vi "Make All Msg.vi"() -> ()   [LabVIEW 2019]
uses:
  00600bcc-c937-488e-a5fa-b30d8be2e7ff.vi
panel:
  out "Horizontal Progress Bar":i32(slide) max=2959 scale=-1.0..1331467.0
  out "size(s)":i32
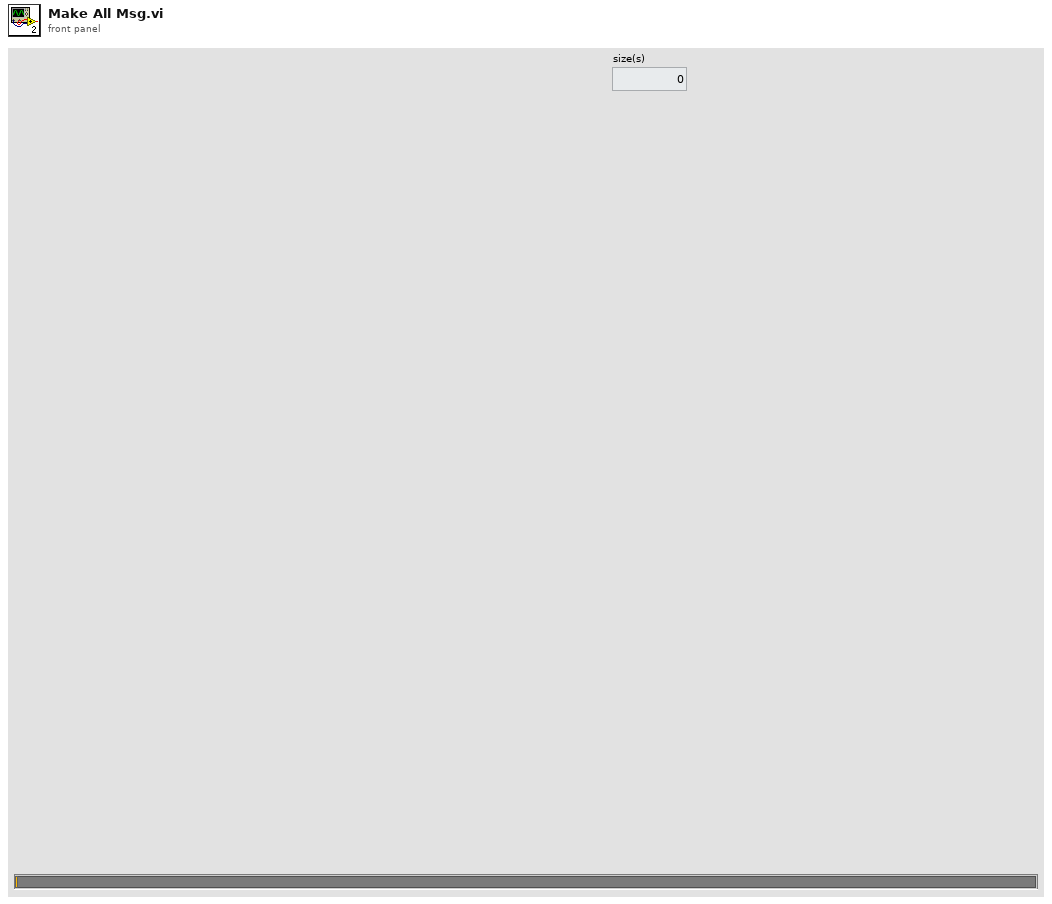
[diagram p1: front panel]
types:
  T1 = enum16{"open", "replace", "create", "open or create", "replace or create", "replace or create with confirmation"}
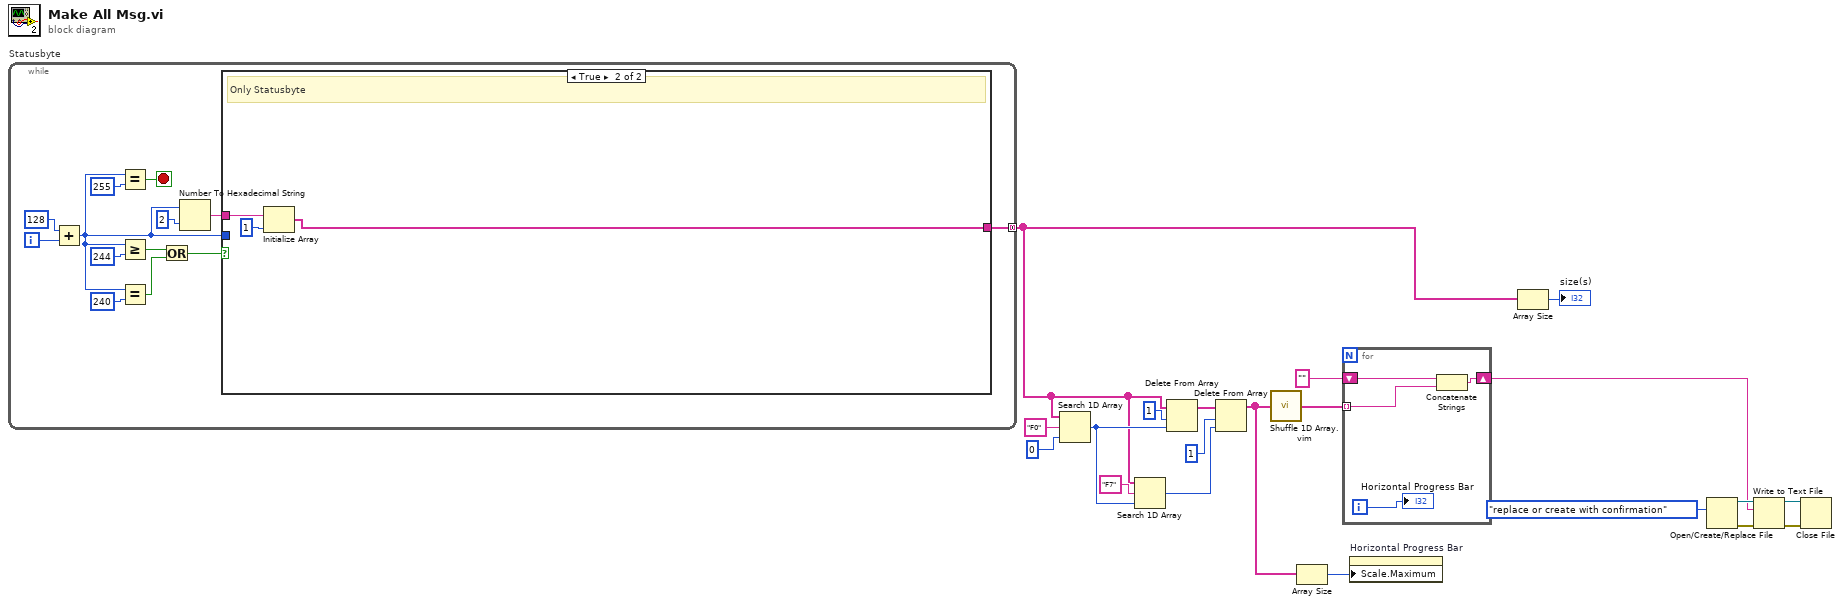
[diagram p0: block diagram]
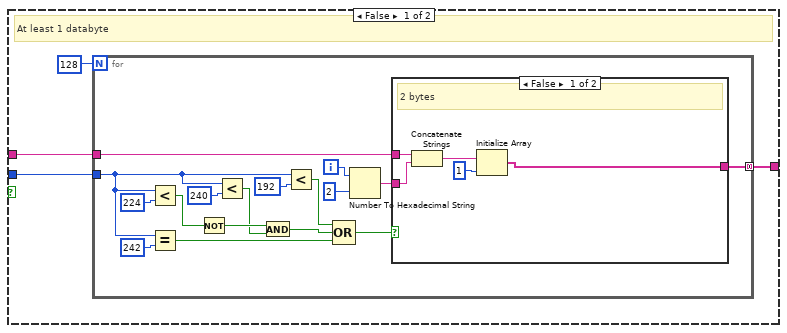
[diagram p2: hidden frame]
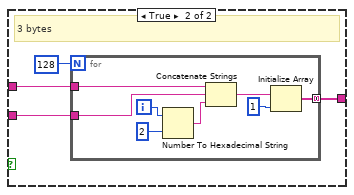
[diagram p3: hidden frame]
diagram:
  n1 = while "Statusbyte" {
    tunnel: [w29] -> w12 mode=concatenating
    i -> [w32]
    stop <- w28 stop-if-true
    n2 = Add(x=128, y=w32) -> (x+y=w23:i32)
    n3 = Equal?(x=w23, y=255) -> (x = y?=w28:bool)
    n4 = Greater Or Equal?(x=w23, y=244) -> (x >= y?=w26:bool)
    n5 = Equal?(x=w23, y=240) -> (x = y?=w21:bool)
    n6 = Or(x=w26, y=w21) -> (x .or. y?=w25:bool)
    n7 = Number To Hexadecimal String(1:i16 2 ("width (-)"), 2:w23) -> (0:w30:string)
    n8 = case shown="True" w25 {
      tunnel: w23 -> [w36 _]
      tunnel: w30 -> [w35 w73]
      tunnel: [w34 w72] -> w29
      frame False {
        # "At least 1 databyte"
        n9 = for {
          N: 128 -> [_]
          tunnel: w36 -> [w44]
          tunnel: w35 -> [w40]
          tunnel: [w38] -> w34 mode=concatenating
          i -> [w41]
          n10 = Less?(x=w44, y=224) -> (x < y?=w54:bool)
          n11 = Equal?(x=w44, y=242) -> (x = y?=w49:bool)
          n12 = Not(x=w54) -> (.not. x?=w53:bool)
          n13 = Less?(x=w44, y=240) -> (x < y?=w52:bool)
          n14 = And(x=w53, y=w52) -> (x .and. y?=w50:bool)
          n15 = Less?(x=w44, y=192) -> (x < y?=w51:bool)
          n16 = Compound Arithmetic op=OR(w51, w50, w49) -> (w43:bool)
          n17 = Number To Hexadecimal String(1:i16 2 ("width (-)"), 2:w41) -> (0:w39:string)
          n18 = case shown="False" w43 {
            tunnel: w40 -> [w57 w62]
            tunnel: w39 -> [w56 w61]
            tunnel: [w55 w60] -> w38
            frame False {
              # "2 bytes"
              n19 = Concatenate Strings(w57, w56) -> (w59:string)
              n20 = Initialize Array(w59, 1 ("dimension size")) -> (w55:string[])
            }
            frame True {
              # "3 bytes"
              n21 = for {
                N: 128 -> [_]
                tunnel: w62 -> [w69]
                tunnel: w61 -> [w68]
                tunnel: [w64] -> w60 mode=concatenating
                i -> [w70]
                n22 = Number To Hexadecimal String(1:i16 2 ("width (-)"), 2:w70) -> (0:w67:string)
                n23 = Concatenate Strings(w69, w68, w67) -> (w66:string)
                n24 = Initialize Array(w66, 1 ("dimension size")) -> (w64:string[])
              }
            }
          }
        }
      }
      frame True {
        # "Only Statusbyte"
        n25 = Initialize Array(w73, 1 ("dimension size")) -> (w72:string[])
      }
    }
  }
  n26 = Search 1D Array(1D array=w12, element="F0", start index (0)=0) -> (index of element=w13:i32)
  n27 = Search 1D Array(1D array=w12, element="F7", start index (0)=w13) -> (index of element=w16:i32)
  n28 = Delete From Array(array=w12, length=1, index=w13) -> (array with subset deleted=w11:string[])  [unwired: 1 out]
  n29 = Delete From Array(array=w11, length=1, index=w16) -> (array with subset deleted=w7:string[])  [unwired: 1 out]
  n30 = call "Shuffle 1D Array.vim"("array"=w7) -> ("shuffled array"=w10:string[])  [unwired: 4 in]
  n31 = Array Size(array=w7) -> (size(s)=w8:i32)
  n32 = for {
    tunnel: w10 -> [w78] mode=indexing
    shift-right: [w76] -> w4
    shift-left: "" -> [w77]
    i -> [w75]
    n33 = Concatenate Strings(w77, w78) -> (w76:string)
    "Horizontal Progress Bar" <- w75
  }
  n34 = property on="Horizontal Progress Bar" class="Slide (strict)"("Scale.Maximum"=w8) -> ()  [unwired: 2 in, 2 out]
  n35 = Array Size(array=w12) -> (size(s)=→"size(s)":i32)
  n36 = Open/Create/Replace File(operation (0:open)=T1."replace or create with confirmation") -> (refnum out=w5:refnum<file>, error out=w6:errorcluster)  [unwired: 5 in, 1 out]
  n37 = Write to Text File(file (use dialog)=w5, text=w4, error in=w6) -> (refnum out=w2:refnum<file>, error out=w3:errorcluster)  [unwired: 1 in, 1 out]
  n38 = Close File(refnum=w2, error in=w3) -> ()  [unwired: 2 out]
